vi "Clear Gameboard.vi"(8 "error in (no error)":errorcluster, 11 "Buton Refs IN":refnum<vi>[](array[refnum])) -> (0 "error out":errorcluster)   [LabVIEW 2020]
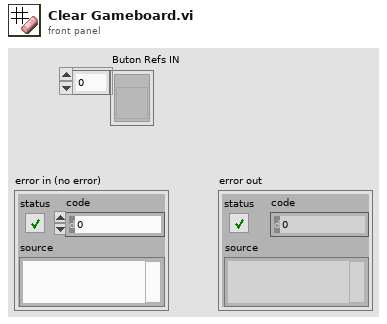
[diagram p1: front panel]
types:
  T1 = enum8{"Enabled", "Disabled", "Disabled and Grayed Out"}
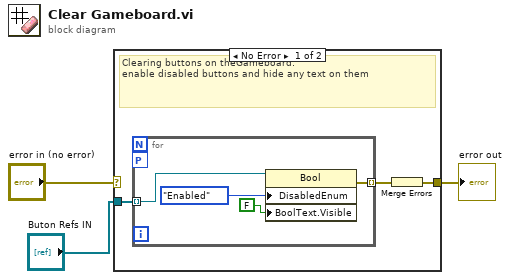
[diagram p0: block diagram]
diagram:
  n1 = case shown="No Error" "error in (no error)" {
    selector: "error in (no error)" -> [_ w11]
    tunnel: "Buton Refs IN" -> [w6 _]
    tunnel: [w4 w11] -> w1
    frame No Error {
      # "Clearing buttons on theGameboard: \nenable disabled buttons and hide any text on them"
      n2 = for {
        tunnel: w6 -> [w10] mode=indexing
        workers-P: _ -> [_]
        tunnel: [w7] -> w5 mode=indexing
        n3 = property class="Bool"(reference=w10, "DisabledEnum"=T1."Enabled" ("Disabled"), "BoolText.Visible"=FALSE ("Boolean Text.Visible")) -> (error out=w7:errorcluster)  [unwired: 1 in, 1 out]
      }
      n4 = Merge Errors(w5) -> (w4:errorcluster)
    }
    frame Error {
    }
  }
  "error out" <- w1
